vi "Write Exported Data Location.vi"(8 "error in (no error)":errorcluster, 10 "Exported Data Location":string, 11 "Harmonics_CHP in":refnum<class "Harmonics_CHP.lvclass">=refnum) -> (0 "error out":errorcluster, 3 "Harmonics_CHP out":refnum<class "Harmonics_CHP.lvclass">)   [LabVIEW 2016, in "SeqAuto Evaluations.lvlib" / "Harmonics_CHP.lvclass"]
uses:
  Harmonics_CHP.lvclass
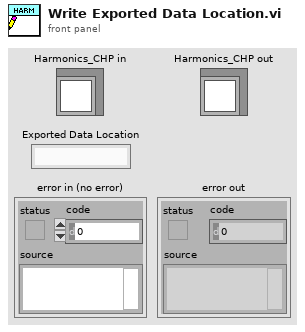
[diagram p1: front panel]
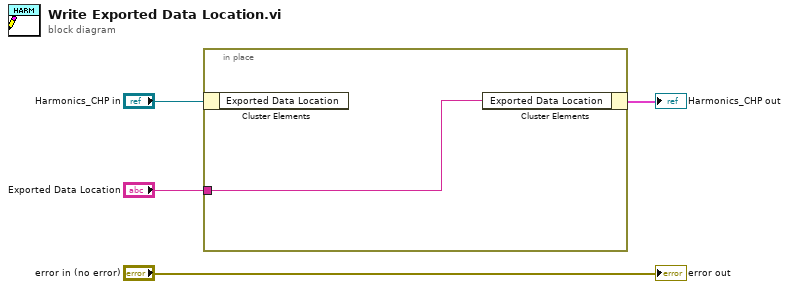
[diagram p0: block diagram]
diagram:
  n1 = in-place {
    in-place-border: "Exported Data Location" -> [w5]
    n2 = in-place-cluster #1("Harmonics_CHP in") -> ()  [unwired: 1 out]
    n3 = in-place-cluster #1("Exported Data Location"=w5) -> (→"Harmonics_CHP out":cluster{})
  }
  "error out" <- "error in (no error)"
